vi "Switch.vi"(8 "Position":T1) -> ()   [LabVIEW 2017]
uses:
  Support Code/Starting Position.ctl
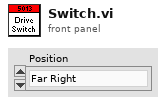
[diagram p1: front panel]
types:
  T1 = typedef "Starting Position.ctl" = enum16{"Far Right", "Far Left"}
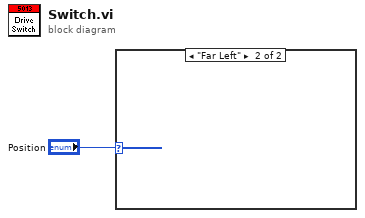
[diagram p0: block diagram]
diagram:
  n1 = case shown="\"Far Left\"" "Position" {
    frame "Far Right" {
    }
    frame "Far Left" {
    }
  }
